vi "Method.vi"(4 "Input B":refnum<class "Abs_Numeric.lvclass">, 5 "Abs_Integer.lvclass":refnum<class "Abs_Integer.lvclass">) -> (1 "Abs_Double Float.lvclass":refnum<class "Abs_Double Float.lvclass">)   [LabVIEW 2021, in "Divide_INT.lvclass"]
uses:
  Divide_INT.lvclass
  Abs_Types/Numeric/Abs_Numeric.lvclass
  Abs_Types/Double Float/Abs_Double Float.lvclass
  Abs_Types/Integer/Abs_Integer.lvclass
  C:/Users/Tim/Documents/LabVIEW/2021/Data Classes/Source/Abs_Types/Double Float/Abs_Double Float.lvclass
  Divide_INT.lvclass/Divide_INT.ctl
  Properties/Write Numeric A.vi
  Properties/Write Numeric B.vi
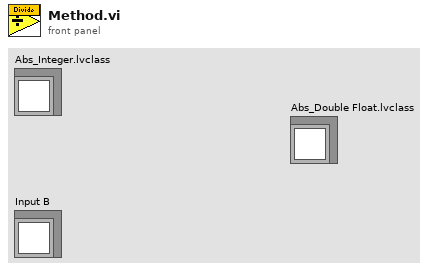
[diagram p1: front panel]
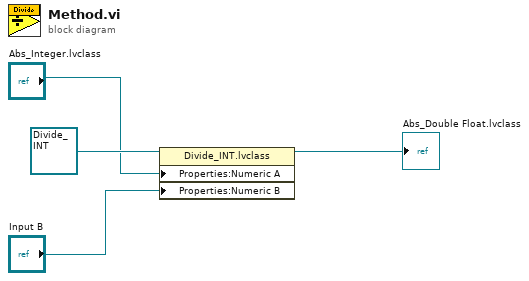
[diagram p0: block diagram]
diagram:
  n1 = property class="Divide_INT.lvclass"(reference=refnum<class "Divide_INT.lvclass"> refnum ("Functions.lvlib:Numeric.lvlib:Divide.lvclass"), "Properties:Numeric A"="Abs_Integer.lvclass", "Properties:Numeric B"="Input B") -> (reference out=→"Abs_Double Float.lvclass":refnum<class "Divide_INT.lvclass">)  [unwired: 1 in, 1 out]
